vi "fgen_arb_scrip.vi"() -> ()   [LabVIEW 2020]
uses:
  <instrlib>/niFgen/niFgen.llb/niFgen_ctl Trigger Script - trigID Values (Ring).ctl
  <instrlib>/niFgen/niFgen.llb/niFgen Output Mode.ctl
  <instrlib>/niFgen/niFgen.llb/niFgen_ctl Trigger DigEdge - Edge Values (Ring).ctl
  <instrlib>/niFgen/niFgen.llb/niFgen_ctl Trigger DigLvl - Level Values (Ring).ctl
  <instrlib>/niFgen/niFgen.llb/niFgen_ctl Trigger SW - TrigName Values (Ring).ctl
  <instrlib>/niFgen/niFgen.llb/niFgen Disable Script Trigger.vi
  <instrlib>/niFgen/niFgen.llb/niFgen Configure Software Edge Script Trigger.vi
  <instrlib>/niFgen/niFgen.llb/niFgen Configure Digital Edge Script Trigger.vi
  <instrlib>/niFgen/niFgen.llb/niFgen Configure Digital Level Script Trigger.vi
  <instrlib>/niFgen/niFgen.llb/niFgen Write Named Waveform (I16).vi
panel:
  in  "Script to Generate":u16(ring) items=["myScript0", "myScript1", "myScript2", "myScript3", "myScript4"]
  in  "Scripts Array":string[](array[string])=["script myScript0\n    Generate wfmSquare\n    Generate wfmSine\n    Generate wfmTriangle\n    Generate wfmSine\n    Generate wfmDC0V\nend script", "script myScript1\n  Wait until scriptTrigger0\n  Generate wfmSquare\n  Generate wfmSine\n  Generate wfmTriangle\n  Generate wfmSine\n  Generate wfmDC0V\nend script", "script myScript2\n  Generate wfmSquare\n  Repeat 2\n    Generate wfmSine\n  end repeat\n  Repeat 5\n    Generate wfmTriangle\n  end repeat\n  Repeat 2\n    Generate wfmSine\n  end repeat\n  Repeat 3\n    Generate wfmDC0V\n  end repeat\nend script", "script myScript3\n  Wait until scriptTrigger0\n  Generate wfmSquare\n  Repeat 2\n    Generate wfmSine\n  end repeat\n  Repeat 5\n    Generate wfmTriangle\n  end repeat\n  Repeat 2\n    Generate wfmSine\n  end repeat\n  Repeat 3\n    Generate wfmDC0V\n  end repeat\nend script", "script myScript4\n  Repeat forever\n    Generate wfmSquare\n    Repeat 2\n      Generate wfmSine\n    end repeat\n    Repeat 5\n      Generate wfmTriangle\n    end repeat\n    Repeat 2\n      Generate wfmSine\n    end repeat\n    Repeat 3\n      Generate wfmDC0V\n    end repeat\n  end repeat\nend script"]
  in  "Script Trigger Source":string(combo)="PFI0"
  in  "Waveform Information Array":T1(array[cluster])=[{"Name"="wfmSine", "Waveform"={"Waveform Type"=0, "Amplitude"=0.5, "# of points"=256}}, {"Name"="wfmSquare", "Waveform"={"Waveform Type"=3, "Amplitude"=1.0, "# of points"=256}}, {"Name"="wfmTriangle", "Waveform"={"Waveform Type"=2, "Amplitude"=0.5, "# of points"=256}}, {"Name"="wfmDC0V", "Waveform"={"Waveform Type"=7, "Amplitude"=0.0, "# of points"=256}}] {"Waveform"."Amplitude" min=0.0 max=1.0 format="%.2f"; "Waveform"."Waveform Type" items=["Sine", "Cosine", "Triangle", "Square", "Sawtooth", "Increasing Ramp", "Decreasing Ramp", "DC Value"]}
  in  "Script Trigger Type":u16(ring) items=["None", "Software Edge", "Digital Edge", "Digital Level"]
  in  "FGEN Resource Name":refnum<k15>
  in  "Stop":bool
  in  "Send Software Trigger":bool
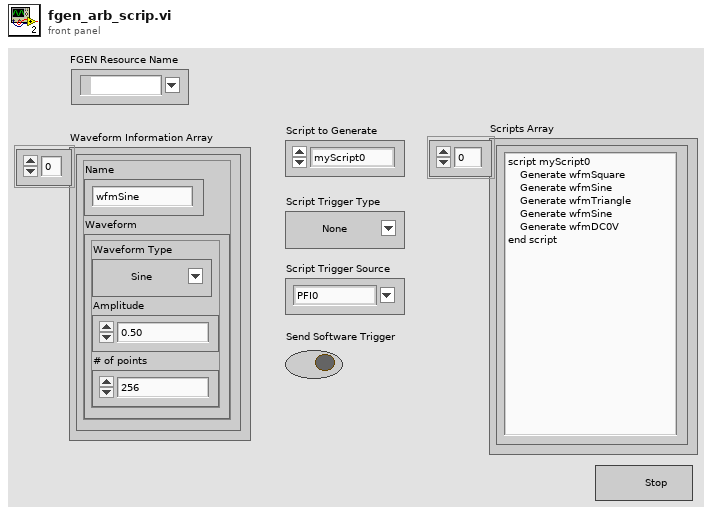
[diagram p1: front panel]
types:
  T1 = cluster{"Name":string, "Waveform":cluster{"Waveform Type":u16, "Amplitude":dbl, "# of points":u32}}[]
  T2 = typedef "niFgen Output Mode.ctl" = u32
  T3 = typedef "niFgen_ctl Trigger Script - trigID Values (Ring).ctl" = string
  T4 = typedef "niFgen_ctl Trigger DigEdge - Edge Values (Ring).ctl" = i32
  T5 = typedef "niFgen_ctl Trigger DigLvl - Level Values (Ring).ctl" = i32
  T6 = cluster{"Waveform Type":u16, "Amplitude":dbl, "# of points":u32}
  T7 = typedef "niFgen_ctl Trigger SW - TrigName Values (Ring).ctl" = i32
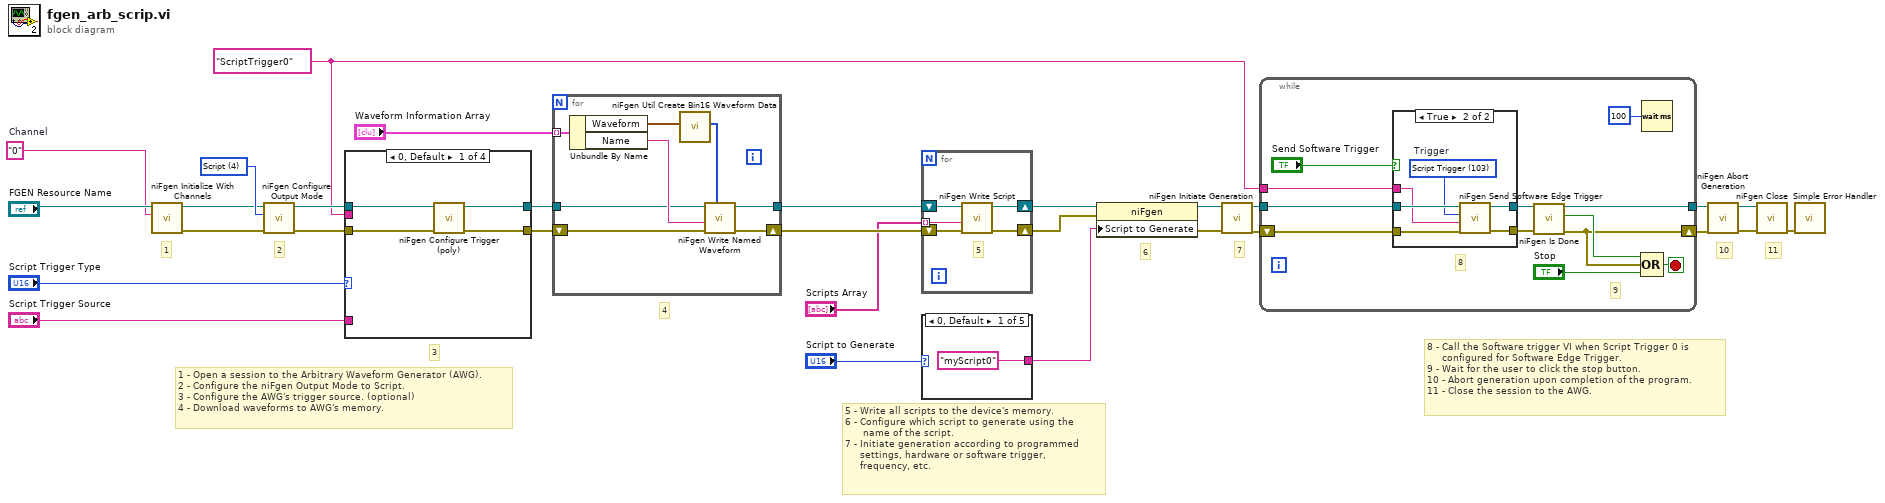
[diagram p0: block diagram]
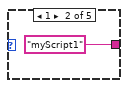
[diagram p2: hidden frame]
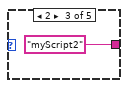
[diagram p3: hidden frame]
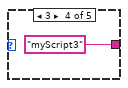
[diagram p4: hidden frame]
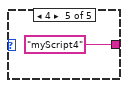
[diagram p5: hidden frame]
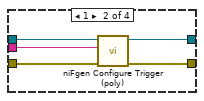
[diagram p6: hidden frame]
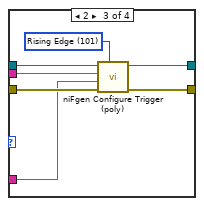
[diagram p7: hidden frame]
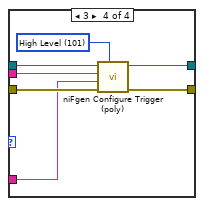
[diagram p8: hidden frame]
diagram:
  w1 = "0"  # Channel
  w15 = T2 4 items=["Standard Function", "Frequency List", "Arbitrary Waveform", "Arbitrary Sequence", "Script"] ("Output Mode")
  w19 = T3 "ScriptTrigger0" ("Trigger ID (Script Trigger 0)")
  # "6"
  # "11"
  # "10"
  # "7"
  # "4"
  # "3"
  # "2"
  # "1"
  # "8 - Call the Software trigger VI when Script Trigger 0 is \n     configured for Software Edge Trigger.\n9 - Wait for the user to click the stop button.\n10 - Abort generation upon completion of the program. \n11 - Close the session to the AWG."
  # "5 - Write all scripts to the device's memory.\n6 - Configure which script to generate using the \n      name of the script.\n7 - Initiate generation according to programmed \n     settings, hardware or software trigger, \n     frequency, etc."
  # "1 - Open a session to the Arbitrary Waveform Generator (AWG).\n2 - Configure the niFgen Output Mode to Script.\n3 - Configure the AWG's trigger source. (optional)\n4 - Download waveforms to AWG's memory."
  n1 = call <instrlib>:"niFgen Initialize With Channels.vi"("Channel Name"=w1, "Resource Name"="FGEN Resource Name") -> ("error out"=w2:errorcluster, "Instrument Handle Out"=w3:refnum<k15>)  [unwired: 8 in]
  n2 = call <instrlib>:"niFgen Configure Output Mode.vi"("error in (no error)"=w2, "Output Mode (default: 0=Standard Function)"=w15, "Instrument Handle"=w3) -> ("error out"=w22:errorcluster, "Instrument Handle Out"=w23:refnum<k15>)  [unwired: 6 in]
  n3 = case shown="0, Default" "Script Trigger Type" {
    tunnel: w23 -> [w33 w38 w45 w52]
    tunnel: w22 -> [w32 w37 w44 w51]
    tunnel: [w31 w36 w43 w50] -> w21
    tunnel: [w30 w35 w42 w49] -> w20
    tunnel: w19 -> [_ w34 w41 w48]
    tunnel: "Script Trigger Source" -> [_ _ w39 w46]
    frame 0, Default {
      n4 = call-poly <instrlib>:"niFgen Configure Trigger (poly).vi"("error in (no error)"=w32, "Instrument Handle"=w33) -> ("error out"=w31:errorcluster, "Instrument Handle Out"=w30:refnum<k15>)  [unwired: 8 in]
    }
    frame 1 {
      n5 = call-poly <instrlib>:"niFgen Configure Trigger (poly).vi"("error in (no error)"=w37, "Trigger ID (Script Trigger 0)"=w34, "Instrument Handle"=w38) -> ("error out"=w36:errorcluster, "Instrument Handle Out"=w35:refnum<k15>)  [unwired: 7 in]
    }
    frame 2 {
      w40 = T4 101 items=["Rising Edge"=101, "Falling Edge"=102] ("Edge (Rising)")
      n6 = call-poly <instrlib>:"niFgen Configure Trigger (poly).vi"("Edge (Rising)"=w40, "error in (no error)"=w44, "Source"=w39, "Trigger ID (Script Trigger 0)"=w41, "Instrument Handle"=w45) -> ("error out"=w43:errorcluster, "Instrument Handle Out"=w42:refnum<k15>)  [unwired: 5 in]
    }
    frame 3 {
      w47 = T5 101 items=["High Level"=101, "Low Level"=102] ("Trigger When (High)")
      n7 = call-poly <instrlib>:"niFgen Configure Trigger (poly).vi"("Trigger When (High)"=w47, "error in (no error)"=w51, "Source"=w46, "Trigger ID (Script Trigger 0)"=w48, "Instrument Handle"=w52) -> ("error out"=w50:errorcluster, "Instrument Handle Out"=w49:refnum<k15>)  [unwired: 5 in]
    }
  }
  n8 = for {
    shift-right: [w57] -> w17
    shift-left: w21 -> [w55]
    tunnel: [w58] -> w18
    tunnel: w20 -> [w54]
    tunnel: "Waveform Information Array" -> [w60] mode=indexing
    n9 = Unbundle By Name(w60) -> ("Waveform"=w53:T6, "Name"=w56:string)
    n10 = call <instrlib>:"niFgen Util Create Bin16 Waveform Data.vi"("Waveform"=w53) -> ("Waveform Data"=w59:i16[])  [unwired: 10 in]
    n11 = call-poly <instrlib>:"niFgen Write Named Waveform.vi"("Waveform Data"=w59, "error in (no error)"=w55, "Waveform Name"=w56, "Instrument Handle"=w54) -> ("error out"=w57:errorcluster, "Instrument Handle Out"=w58:refnum<k15>)  [unwired: 5 in, 1 out]
  }
  n12 = for {
    shift-right: [w62] -> w9
    shift-left: w18 -> [w65]
    shift-right: [w63] -> w16
    shift-left: w17 -> [w64]
    tunnel: "Scripts Array" -> [w61] mode=indexing
    # "5"
    n13 = call <instrlib>:"niFgen Write Script.vi"("error in (no error)"=w64, "Script"=w61, "Instrument Handle"=w65) -> ("error out"=w63:errorcluster, "Instrument Handle Out"=w62:refnum<k15>)  [unwired: 7 in]
  }
  n14 = case shown="0, Default" "Script to Generate" {
    tunnel: ["myScript0" "myScript1" "myScript2" "myScript3" "myScript4"] -> w5
    frame 0, Default {
    }
    frame 1 {
    }
    frame 2 {
    }
    frame 3 {
    }
    frame 4 {
    }
  }
  n15 = property class="niFgen"(reference=w9, error in=w16, "Script to Generate"=w5) -> (reference out=w8:refnum<k15>, error out=w10:errorcluster)
  n16 = call <instrlib>:"niFgen Initiate Generation.vi"("error in (no error)"=w10, "Instrument Handle"=w8) -> ("error out"=w26:errorcluster, "Instrument Handle Out"=w27:refnum<k15>)  [unwired: 8 in]
  n17 = while {
    tunnel: w27 -> [w82]
    tunnel: [w75] -> w25
    tunnel: w19 -> [w80]
    shift-right: [w71] -> w24
    shift-left: w26 -> [w81]
    stop <- w79 stop-if-true
    # "9"
    # "8"
    n18 = case shown="True" "Send Software Trigger" {
      tunnel: w82 -> [w84 w90]
      tunnel: w81 -> [w83 w89]
      tunnel: [w83 w88] -> w77
      tunnel: [w84 w87] -> w78
      tunnel: w80 -> [_ w85]
      frame False {
      }
      frame True {
        w86 = T7 103 items=["Start Trigger"=1004, "Script Trigger"=103]  # Trigger
        n19 = call <instrlib>:"niFgen Send Software Edge Trigger.vi"("error in (no error)"=w89, "Trigger ID (None)"=w85, "Trigger (Start Trigger)"=w86, "Instrument Handle"=w90) -> ("error out"=w88:errorcluster, "Instrument Handle Out"=w87:refnum<k15>)  [unwired: 6 in]
      }
    }
    n20 = call <instrlib>:"niFgen Is Done.vi"("error in (no error)"=w77, "Instrument Handle"=w78) -> ("error out"=w71:errorcluster, "Done"=w76:bool, "Instrument Handle Out"=w75:refnum<k15>)  [unwired: 7 in]
    n21 = Compound Arithmetic op=OR(w76, w71, "Stop") -> (w79:bool)
    n22 = Wait (ms)(milliseconds to wait=u32 100 ("millisecond multiple")) -> ()  [unwired: 1 out]
  }
  n23 = call <instrlib>:"niFgen Abort Generation.vi"("error in (no error)"=w24, "Instrument Handle"=w25) -> ("error out"=w28:errorcluster, "Instrument Handle Out"=w29:refnum<k15>)  [unwired: 8 in]
  n24 = call <instrlib>:"niFgen Close.vi"("error in (no error)"=w28, "Instrument Handle"=w29) -> ("error out"=w12:errorcluster)  [unwired: 9 in]
  n25 = call <vilib>:"Simple Error Handler.vi"("error in (no error)"=w12) -> ()  [unwired: 4 in, 5 out]
